vi "Post_process.vi"() -> ()   [LabVIEW 2020]
uses:
  <vilib>/Platform/NI_3dgraph.lvlib
panel:
  out "channel name(s) out":string[](array[string])
  out "data":dbl[][](array[numeric])
  in  "3D Surface":refnum<k7>(container)
  out "Latest Spectrum":cluster{"WavelengthCal":dbl[], "Array":i32[]}(graph)
  out "Chromatogram at wavelength of interest":i32[](graph)
  in  "Length of Chromatogram (sec)":dbl=120.0
  in  "Wavelength of Interest (nm)":dbl=500.0
  in  "Date file path":path
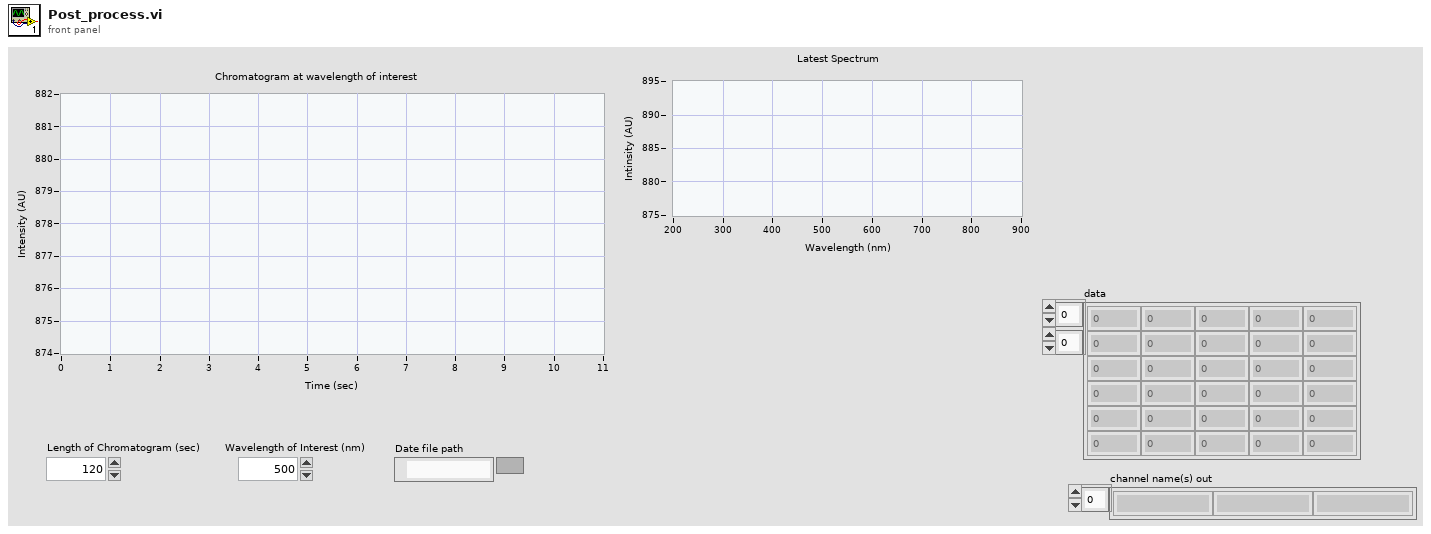
[diagram p1: front panel]
types:
  T1 = enum16{"open", "open or create", "create or replace", "create", "open (read-only)"}
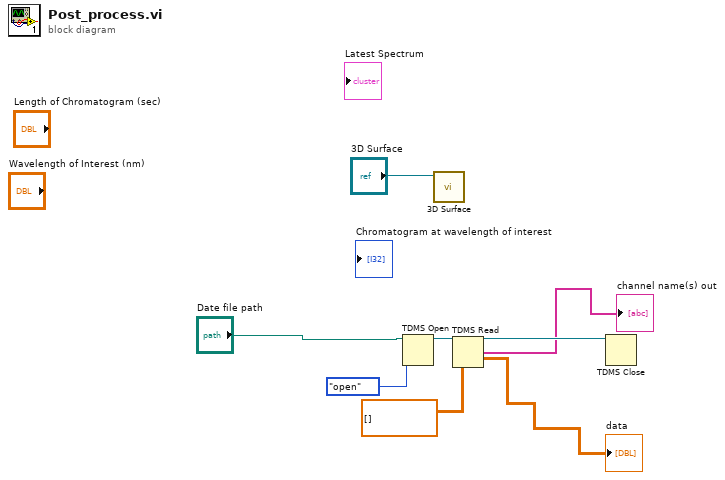
[diagram p0: block diagram]
diagram:
  n1 = TDMS Open(10:T1."open" ("operation (0:open)"), 11:"Date file path") -> (3:w8:refnum<k34>)  [unwired: 5 in, 1 out]
  n2 = call <vilib>:"3D Surface.vi"("3D graph"="3D Surface") -> ()  [unwired: 9 in, 2 out]
  n3 = TDMS Read(0:w8, 12:dbl[][] []) -> (4:w7:refnum<k34>, 8:→"channel name(s) out":string[], 10:→"data":dbl[][])  [unwired: 6 in, 3 out]
  n4 = TDMS Close(11:w7) -> ()  [unwired: 1 in, 2 out]
